vi "User_list.vi"(3 "error in (no error)":errorcluster, 5 "连接模式":enum16{"单机", "联网"}(ring)) -> (0 "错误输出":errorcluster, 2 "User_list":cluster{string, string}[](array[cluster]))   [LabVIEW 2020]
uses:
  <vilib>/addons/database/Connection.llb/DB Tools Open Connec (String).vi
  <vilib>/addons/database/Connection.llb/Conn Execute.vi
  <vilib>/addons/database/Recordset.llb/Rec Fetch Recordset Data (R).vi
  <vilib>/addons/database/Recordset.llb/Rec Destroy - Connection.vi
  <vilib>/addons/database/NI_Database_API.lvlib
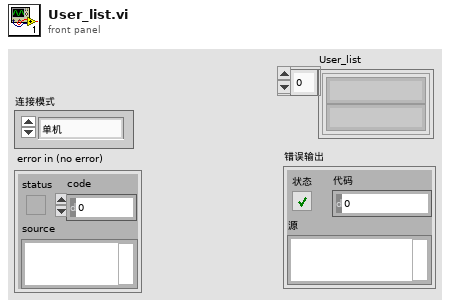
[diagram p1: front panel]
types:
  T1 = typedef "NI_Database_API.lvlib/Conn ObjectReference.ctl" = refnum<k1>
  T2 = typedef "NI_Database_API.lvlib/Rec ObjectReference.ctl" = refnum<k1>
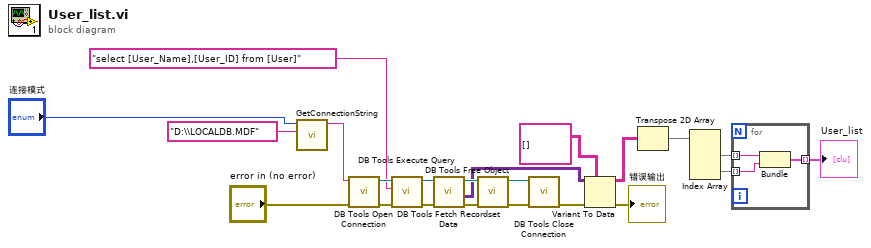
[diagram p0: block diagram]
diagram:
  n1 = call "GetConnectionString.vi"("Database Name"="D:\\LOCALDB.MDF", "连接模式"="连接模式") -> ("连接字符串"=w21:string)  [unwired: 4 in, 1 out]
  n2 = call-poly <vilib>:"DB Tools Open Connection.vi"("error in (no error)"="error in (no error)", "connection information"=w21) -> ("error out"=w20:errorcluster, "connection reference"=w19:T1)  [unwired: 6 in]
  n3 = call-poly <vilib>:"DB Tools Execute Query.vi"("error in (no error)"=w20, "SQL query"="select [User_Name],[User_ID] from [User]", "connection reference"=w19) -> ("error out"=w14:errorcluster, "recordset reference"=w16:T2)  [unwired: 5 in]
  n4 = call-poly <vilib>:"DB Tools Fetch Recordset Data.vi"("error in (no error)"=w14, "recordset reference"=w16) -> ("error out"=w13:errorcluster, "recordset data"=w11:variant[][], "recordset reference out"=w15:T2)  [unwired: 3 in]
  n5 = call-poly <vilib>:"DB Tools Free Object.vi"("error in (no error)"=w13, "recordset reference"=w15) -> ("error out"=w18:errorcluster, "connection reference"=w17:T1)  [unwired: 8 in]
  n6 = call <vilib>:"DB Tools Close Connection.vi"("error in (no error)"=w18, "connection reference"=w17) -> ("error out"=w12:errorcluster)  [unwired: 5 in]
  n7 = Variant To Data(error in=w12, type=string[][] [], Variant=w11) -> (data=w8:string[][], error out=→"错误输出":errorcluster)
  n8 = Transpose 2D Array(2D array=w8) -> (transposed array=w7:string[][])
  n9 = Index Array(array=w7) -> (element #1=w4:string[], element #2=w3:string[])  [unwired: 4 in]
  n10 = for {
    tunnel: w4 -> [w25] mode=indexing
    tunnel: w3 -> [w24] mode=indexing
    tunnel: [w23] -> w2 mode=indexing
    n11 = Bundle(w25, w24) -> (w23:cluster{string, string})  [unwired: 1 in]
  }
  "User_list" <- w2
